vi "Append File to Report.vi"(0 "report in":refnum<class "NI_Excel.lvclass">, 1 "MS Office parameters":T1, 7 "file path":path, 9 "is spreadsheet file? (Excel)":bool, 11 "error in (no error)":errorcluster) -> (4 "report out":refnum<class "NI_Excel.lvclass">, 8 "start out (Word)":i32, 10 "end out (Word)":i32, 15 "error out":errorcluster)   [LabVIEW 2020, in "NI_Excel.lvclass"]
doc: "Appends the text from a text file into the current report."
uses:
  <vilib>/Utility/NIReport.llb/Excel/NI_Excel.lvclass
  <vilib>/Utility/NIReport.llb/Excel/NI_Excel.lvclass/NI_Excel.ctl
  <vilib>/addons/_office/NI_ReportGenerationToolkit.lvlib
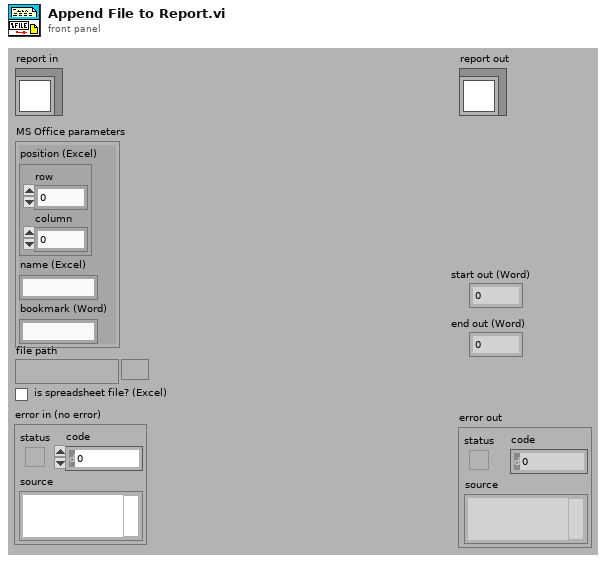
[diagram p1: front panel]
types:
  T1 = cluster{"position (Excel)":cluster{"row":i32, "column":i32}, "name (Excel)":string, "bookmark (Word)":string}
  T2 = typedef "NI_ReportGenerationCore.lvlib/Report Data Members.ctl" = cluster{"font":T3, "from template?":bool}
  T3 = typedef "NI_ReportGenerationCore.lvlib/font.ctl" = cluster{"font name":string, "font size":dbl, "bold":u16, "italic":u16, "underline":u16, "strike through":u16, "font color":u32}
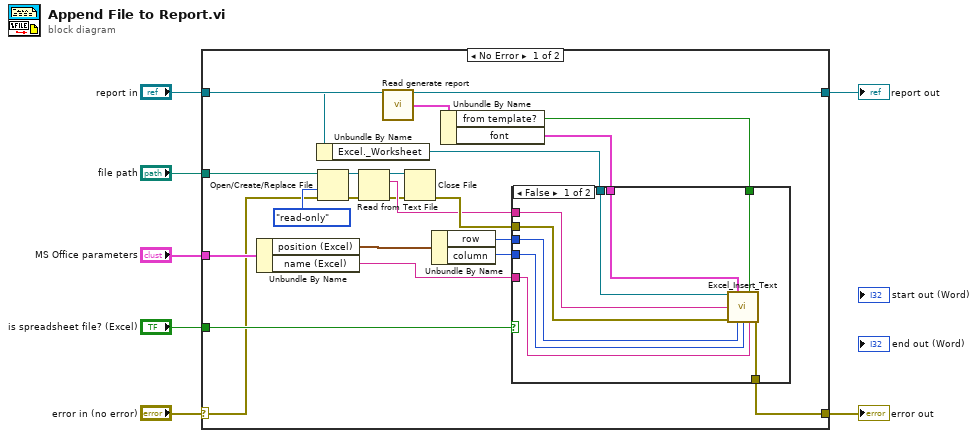
[diagram p0: block diagram]
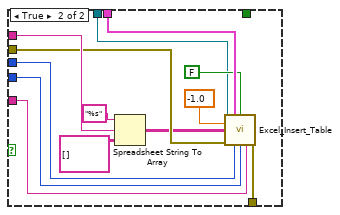
[diagram p2: hidden frame]
diagram:
  n1 = case shown="No Error" "error in (no error)" {
    selector: "error in (no error)" -> [w14 w53]
    tunnel: [w13 w53] -> w6
    tunnel: [w11 w52] -> w4
    tunnel: "report in" -> [w12 w52]
    tunnel: "is spreadsheet file? (Excel)" -> [w17 _]
    tunnel: "MS Office parameters" -> [w16 _]
    tunnel: "file path" -> [w15 _]
    frame No Error {
      n2 = Unbundle By Name(w16) -> ("position (Excel)"=w18:cluster{"row":i32, "column":i32}, "name (Excel)"=w19:string)
      n3 = Open/Create/Replace File(file path (use dialog)=w15, error in=w14, access (0:read/write)=enum16{"read/write", "read-only", "write-only"}."read-only") -> (refnum out=w25:refnum<file>, error out=w24:errorcluster)  [unwired: 4 out]
      n4 = Read from Text File(file (use dialog)=w25, error in=w24) -> (refnum out=w26:refnum<file>, text=w28:string, error out=w27:errorcluster)  [unwired: 3 out]
      n5 = call-dynamic "Read generate report.vi"("report in"=w12) -> ("report out"=w11:refnum<class "NI_Excel.lvclass">, "generate report"=w10:T2)  [unwired: 12 in, 1 out]
      n6 = Unbundle By Name(w11) -> ("Excel._Worksheet"=w20:refnum<k7>)
      n7 = Close File(refnum=w26, error in=w27) -> (error out=w29:errorcluster)  [unwired: 1 out]
      n8 = Unbundle By Name(w18) -> ("row"=w21:i32, "column"=w22:i32)
      n9 = Unbundle By Name(w10) -> ("from template?"=w9:bool, "font"=w8:T3)
      n10 = case shown="False" w17 {
        tunnel: w20 -> [w34 w41]
        tunnel: w8 -> [w32 w44]
        tunnel: w21 -> [w36 w46]
        tunnel: w22 -> [w37 w47]
        tunnel: w29 -> [w31 w45]
        tunnel: w28 -> [w35 w51]
        tunnel: w19 -> [w38 w48]
        tunnel: w9 -> [w33 _]
        tunnel: [w30 w39] -> w13
        frame False {
          n11 = call <vilib>:"Excel_Insert_Text.vi"("worksheet"=w34, "font"=w32, "from template?"=w33, "value"=w35, "error in (no error)"=w31, "row"=w36, "column"=w37, "name"=w38) -> ("error out"=w30:errorcluster)  [unwired: 7 out]
        }
        frame True {
          n12 = Spreadsheet String To Array(format string="%s", spreadsheet string=w51, array type (2D Dbl)=string[][] [] ("Array Constant")) -> (array=w42:string[][])  [unwired: 1 out]
          n13 = call <vilib>:"Excel_Insert_Table.vi"("worksheet"=w41, "font"=w44, "show grid lines"=FALSE, "column width (1)"=-1.0, "table"=w42, "error in (no error)"=w45, "Start row"=w46, "Start column"=w47, "name"=w48) -> ("error out"=w39:errorcluster)  [unwired: 1 in, 5 out]
        }
      }
    }
    frame Error {
    }
  }
  "error out" <- w6
  "report out" <- w4
